vi "Obtain Session.vi"(5 "Name":string, 7 "Description":string, 9 "Unit":string, 11 "error in (no error)":errorcluster) -> (4 "Session Handle":T1, 15 "error out":errorcluster)   [LabVIEW 2020, in "Metric Session.lvclass"]
doc: "This function initializes the measurement\n\nPass the function a name to obtain an active measurement handle"
uses:
  Metric Session.lvclass
  Typedefs/Session Handle.ctl
  C:/Program Files (x86)/National Instruments/LabVIEW 2020/user.lib/_Session Fwk/Session - Root.lvclass
  Metric Session.lvclass/Metric Session.ctl
  <userlib>/_Session Fwk/Session - Root.lvclass
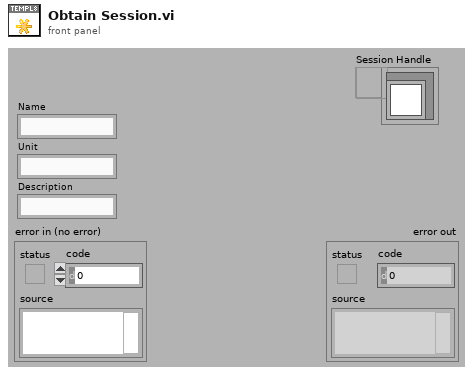
[diagram p1: front panel]
types:
  T1 = typedef "Metric Session.lvclass/Session Handle.ctl" = refnum<data-value>
  T2 = typedef "Session - Root.lvclass/Session Handle.ctl" = refnum<data-value>
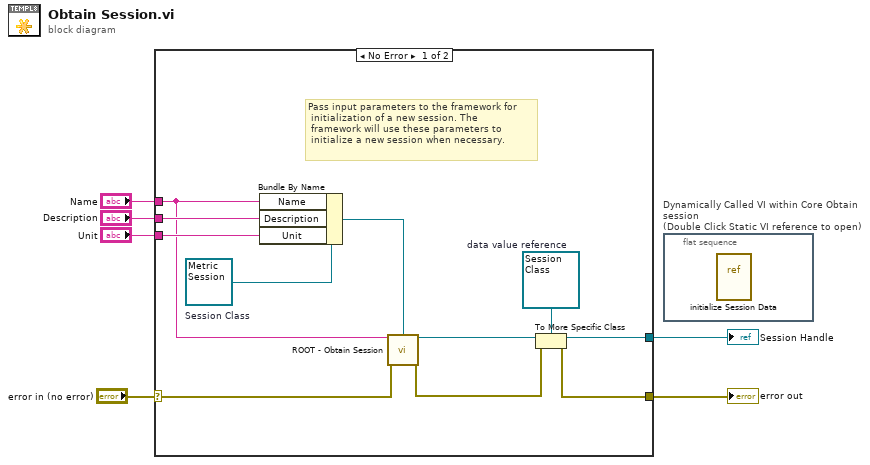
[diagram p0: block diagram]
diagram:
  n1 = case shown="No Error" "error in (no error)" {
    selector: "error in (no error)" -> [w17 w18]
    tunnel: [w14 w18] -> w5
    tunnel: [w16 _] -> w4
    tunnel: "Unit" -> [w9 _]
    tunnel: "Description" -> [w8 _]
    tunnel: "Name" -> [w7 _]
    frame No Error {
      w10 = refnum<data-value> refnum  # data value reference
      w11 = refnum<class "Metric Session.lvclass"> refnum  # Session Class
      # "Pass input parameters to the framework for\n initialization of a new session. The\n framework will use these parameters to\n initialize a new session when necessary."
      n2 = Bundle By Name(cluster=w11, "Name"=w7, "Description"=w8, "Unit"=w9) -> (w12:refnum<class "Metric Session.lvclass">)
      n3 = call <userlib>:"ROOT - Obtain Session.vi"("Session Name ()"=w7, "OBJ - Session"=w12, "error in (no error)"=w17) -> ("Session Handle"=w13:T2, "error out"=w15:errorcluster)  [unwired: 10 in, 1 out]
      n4 = To More Specific Class(target class=w10, reference=w13, error in=w15) -> (specific class reference=w16:refnum<data-value>, error out=w14:errorcluster)
    }
    frame Error {
    }
  }
  "error out" <- w5
  "Session Handle" <- w4
  n5 = flat-sequence "Dynamically Called VI within Core Obtain session\n(Double Click Static VI reference to open)" {
    frame #0 {
      n6 = vi-ref "initialize Session Data.vi"() -> ()  [unwired: 1 out]
    }
  }
